vi "AddDesignPattern.vi"(0 "ClassWriter.lvclass":refnum<class "ClassWriter.lvclass">, 1 "ClassItemRefIn":refnum<vi>, 2 "AddDesignPatternData":T1, 5 "error in (no error)":errorcluster) -> (14 "ClassWriter.lvclass":refnum<class "ClassWriter.lvclass">, 15 "ClassItemRefOut":refnum<vi>, 19 "error out":errorcluster)   [LabVIEW 2016, in "ClassWriter.lvclass"]
uses:
  <resource>/Framework/Providers/Open_GDS/ClassProviders/Provider_BaseClassInterface/ClassWriter_class/ClassWriter.lvclass
  <resource>/Framework/Providers/Open_GDS/ClassProviders/Provider_BaseClassInterface/AddDesignPatternData.ctl
  <resource>/Framework/Providers/Open_GDS/ClassProviders/Common/LvClass_class/GDSLvClass_PlugIn.ctl
  <resource>/Framework/Providers/Open_GDS/ClassProviders/Common/LvClass_class/GDSLvClass_PlugInTypes.ctl
  <resource>/Framework/Providers/Open_GDS/ClassProviders/Provider_BaseClassInterface/BaseProvider_SubVIs/BaseProvider_DesignPatternsActions.ctl
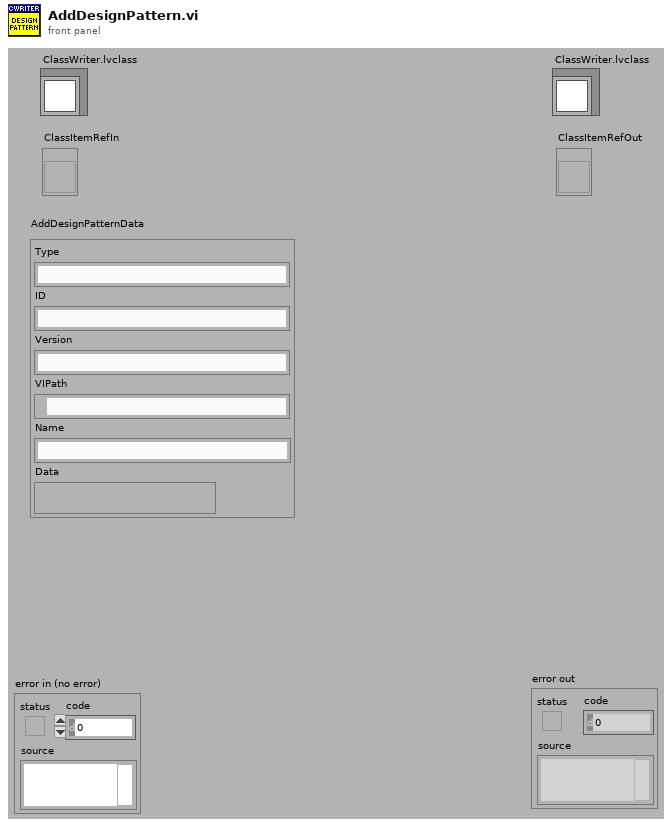
[diagram p1: front panel]
types:
  T1 = typedef "AddDesignPatternData.ctl" = cluster{"Type":string, "ID":string, "Version":string, "VIPath":path, "Name":string, "Data":variant}
  T2 = typedef "GDSLvClass_PlugIn.ctl" = cluster{"Type":T3, "ID":string, "Version":string, "Path":path, "Name":string, "Data":variant}
  T3 = typedef "GDSLvClass_PlugInTypes.ctl" = enum16{"DesignPattern", "MethodTypes"}
  T4 = typedef "BaseProvider_DesignPatternsActions.ctl" = enum16{"AddPatternDialog", "GeneratePattern", "RemovePattern", "CreatePatternMethod", "UpdatePattern"}
  T5 = typedef "GDSLvCLass_ClassSettingsType.ctl" = cluster{"ClassProviderName":string, "ClassTemplateUsed":string, "ClassTemplateVersion":string, "ClassDescription":string, "PlugIns":T2[], "ConnectorPanePattern":string}
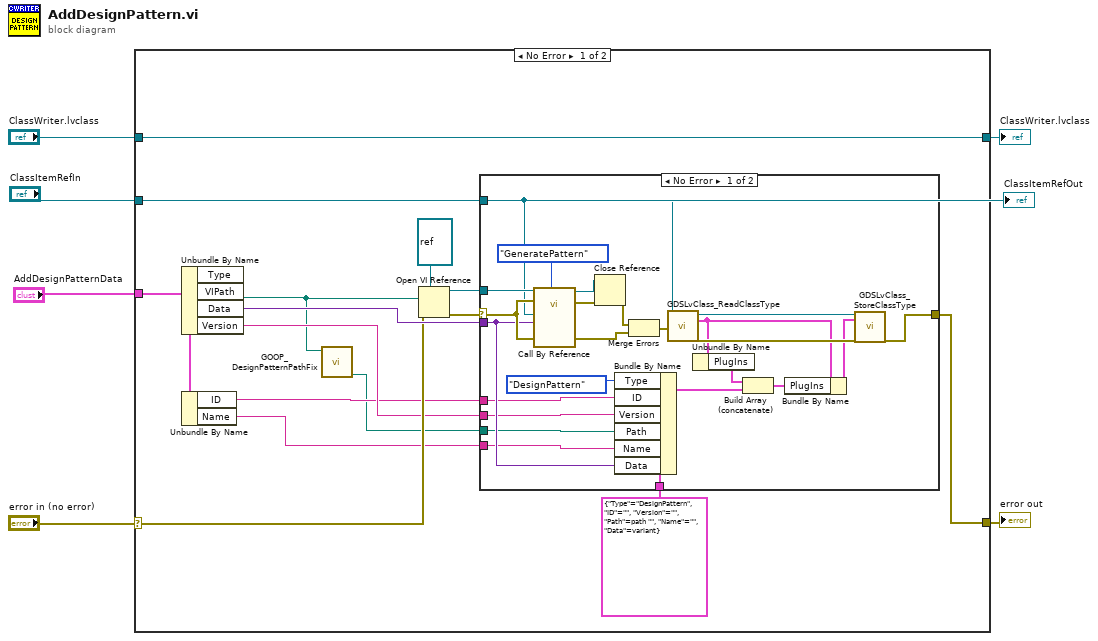
[diagram p0: block diagram]
diagram:
  n1 = case shown="No Error" "error in (no error)" {
    selector: "error in (no error)" -> [w16 w47]
    tunnel: "ClassWriter.lvclass" -> [w21 w48]
    tunnel: [w15 w47] -> w5
    tunnel: [w21 w48] -> w4
    tunnel: "AddDesignPatternData" -> [w12 _]
    tunnel: "ClassItemRefIn" -> [w14 _]
    frame No Error {
      n2 = Unbundle By Name(w12) -> ("VIPath"=w8:path, "Data"=w17:variant, "Version"=w11:string)  [unwired: 1 out]
      n3 = Unbundle By Name(w12) -> ("ID"=w10:string, "Name"=w9:string)
      n4 = call <resource>:"GOOP_DesignPatternPathFix.vi"("ViPathIn"=w8) -> ("RelativeVIPathOut(ToStoreInLvClass)"=w7:path)  [unwired: 6 in, 4 out]
      n5 = Open VI Reference(type specifier VI Refnum (for type only)=refnum<vi> refnum, vi path=w8, error in (no error)=w16) -> (vi reference=w19:refnum<vi>, error out=w18:errorcluster)  [unwired: 3 in]
      n6 = case shown="No Error" w18 {
        selector: w18 -> [w42 w46]
        tunnel: w19 -> [w45 _]
        tunnel: w17 -> [w30 _]
        tunnel: [w39 w46] -> w15
        tunnel: w14 -> [w38 _]
        tunnel: T2 {"Type"=enum."DesignPattern", "ID"="", "Version"="", "Path"=path "", "Name"="", "Data"=variant} ("PlugIn") -> [w33 _]
        tunnel: w7 -> [w27 _]
        tunnel: w10 -> [w28 _]
        tunnel: w11 -> [w26 _]
        tunnel: w9 -> [w22 _]
        frame No Error {
          n7 = call-by-ref "?"(reference=w45, error in=w42, "Action"=BaseProvider_DesignPatternsActions."GeneratePattern", 8:"error in (no error)"=w42, "DataIn"=w30, "ClassRefToActOn"=w38) -> (reference out=w43:refnum<vi>, error out=w44:errorcluster, 0:"error out"=w25:errorcluster)  [unwired: 4 in, 3 out]
          n8 = Close Reference(reference=w43, error in (no error)=w44) -> (error out=w24:errorcluster)
          n9 = Bundle By Name(cluster=w33, "Type"=GDSLvClass_PlugInTypes."DesignPattern", "ID"=w28, "Version"=w26, "Path"=w27, "Name"=w22, "Data"=w30) -> (w32:T2)
          n10 = Merge Errors(w24, w25) -> (w23:errorcluster)
          n11 = call <resource>:"GDSLvClass_ReadClassType.vi"("Class Refnum In"=w38, "error in (no error)"=w23) -> ("Class Refnum Out"=w41:refnum<vi>, "ClassSettings"=w36:T5, "error out"=w40:errorcluster)  [unwired: 15 in]
          n12 = Unbundle By Name(w36) -> ("PlugIns"=w35:T2[])
          n13 = Build Array (concatenate)(w35, w32) -> (w34:T2[])
          n14 = Bundle By Name(cluster=w36, "PlugIns"=w34) -> (w37:T5)
          n15 = call <resource>:"GDSLvClass_StoreClassType.vi"("Class Refnum In"=w41, "ClassSettings"=w37, "error in (no error)"=w40) -> ("error out"=w39:errorcluster)  [unwired: 15 in, 1 out]
        }
        frame Error {
        }
      }
    }
    frame Error {
    }
  }
  "ClassWriter.lvclass" <- w4
  "error out" <- w5
  "ClassItemRefOut" <- "ClassItemRefIn"
